vi "Finish.vi"(8 "error in (no error)":errorcluster, 11 "FormulaG App in":refnum<class "FormulaG App.lvclass">) -> (0 "error out":errorcluster, 3 "FormulaG App out":refnum<class "FormulaG App.lvclass">)   [LabVIEW 2024, in "FormulaG.lvlib" / "FormulaG App.lvclass"]
uses:
  FormulaG App.lvclass
  FormulaG App.lvclass/FormulaG App.ctl
  0cc13077-5977-4511-9e12-66e3febd2798.vi
  Pause Cmd/Pause Cmd.lvclass
  <vilib>/IlluminatedG/IG OBS API/obs-websocket/OBS/OBS.lvclass
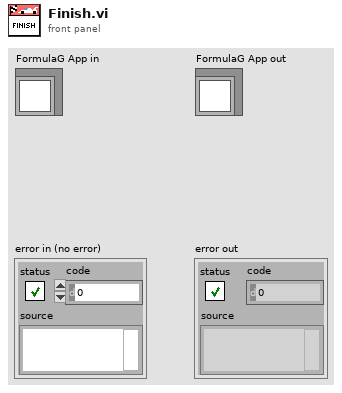
[diagram p1: front panel]
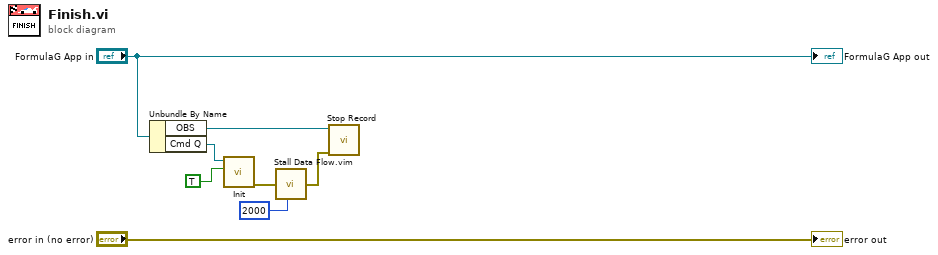
[diagram p0: block diagram]
diagram:
  n1 = Unbundle By Name("FormulaG App in") -> ("OBS"=w2:refnum<class "OBS.lvclass">, "Cmd Q"=w7:refnum<queue>)
  n2 = call "Init.vi"("Pause"=TRUE, "Cmd Q"=w7) -> ("error out"=w4:errorcluster)  [unwired: 9 in]
  n3 = call "Stall Data Flow.vim"("value in"=w4, "milliseconds to wait"=u32 2000) -> ("value out"=w1:errorcluster)  [unwired: 1 out]
  n4 = call <vilib>:"Stop Record.vi"("error in (no error)"=w1, "OBS in"=w2) -> ()  [unwired: 7 in, 3 out]
  "error out" <- "error in (no error)"
  "FormulaG App out" <- "FormulaG App in"
